vi "[PC]Main.vi"() -> ()   [LabVIEW 2018]
panel:
  in  "Kaffee anfordern":bool
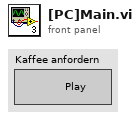
[diagram p1: front panel]
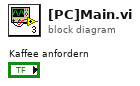
[diagram p0: block diagram]
diagram:
